vi "Single Operation Register Enable.vi"(8 "error in":errorcluster, 9 "Enable":i32 format="%.0x", 11 "Instrument Handle In":i32) -> (0 "error out":errorcluster, 3 "Instrument Handle Out":i32)   [LabVIEW 8.6, in "ZTScopeM.lvlib"]
doc: "Configure the operation status register event forwarding state."
uses:
  ZTScopeM.lvlib
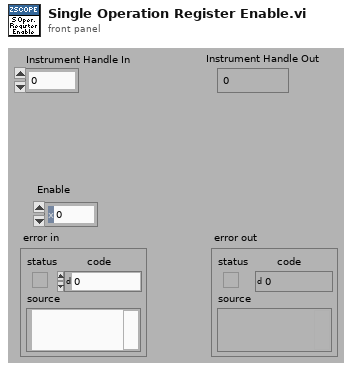
[diagram p1: front panel]
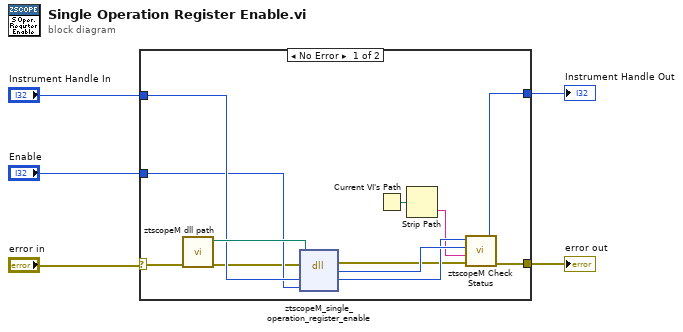
[diagram p0: block diagram]
diagram:
  n1 = case shown="No Error" "error in" {
    selector: "error in" -> [w11 w19]
    tunnel: [w12 w19] -> w4
    tunnel: [w13 w18] -> w3
    tunnel: "Instrument Handle In" -> [w9 w18]
    tunnel: "Enable" -> [w8 _]
    frame #0 {
      n2 = call "ztscopeM dll path.vi"("error in (no error)"=w11) -> ("error out"=w7:errorcluster, "<instrument>.dll path"=w10:path)  [unwired: 9 in]
      n3 = dll-call lib="C:/Program Files (x86)/National Instruments/LabVIEW 2013/instr.lib/ztscopem/ztscopeM.dll" fn="ztscopeM_single_operation_register_enable"(path in=w10, error in=w7, "instrumentHandle"=w9, "enable"=w8) -> (error out=w6:errorcluster, w17:i32, "instrumentHandle"=w16:i32)  [unwired: 2 in, 1 out]
      n4 = Current VI's Path() -> (path=w15:path)
      n5 = Strip Path(path=w15) -> (name=w14:string)  [unwired: 1 out]
      n6 = call "ztscopeM Check Status.vi"("error in"=w6, "name of VI"=w14, "status (return code)"=w17, "instrument handle in"=w16) -> ("error out"=w12:errorcluster, "instrument handle out"=w13:i32)  [unwired: 2 out]
    }
    frame #1 {
    }
  }
  "Instrument Handle Out" <- w3
  "error out" <- w4
